vi "ciclos2.vi"() -> ()   [LabVIEW 2013]
panel:
  out "Menor":dbl
  out "Mayor":dbl
  out "Promedio":dbl
  out "Temperatura":i32(slide) scale=0.0..60.0
  # "Generar 10 temperaturas , y al final presentar la temperatura mayor , menor y la temperatura promedio"
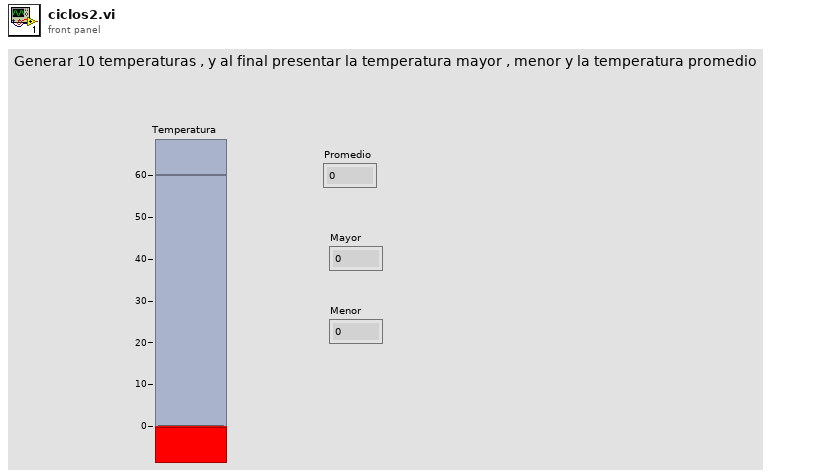
[diagram p1: front panel]
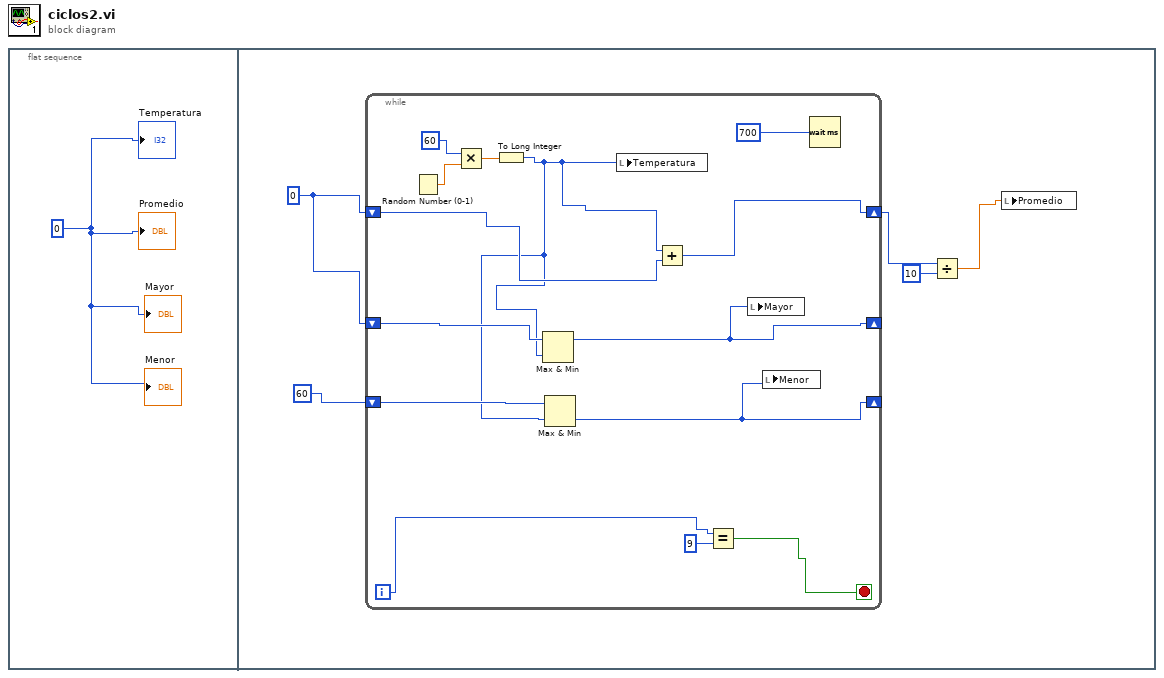
[diagram p0: block diagram]
diagram:
  n1 = flat-sequence {
    frame #0 {
      w1 = 0
      "Temperatura" <- w1
      "Promedio" <- w1
      "Mayor" <- w1
      "Menor" <- w1
    }
    frame #1 {
      w3 = 0
      n2 = while {
        shift-right: [w13] -> w6
        shift-left: w3 -> [w14]
        shift-right: [w8] -> _
        shift-left: w3 -> [w11]
        shift-right: [w7] -> _
        shift-left: 60 -> [w10]
        i -> [w20]
        stop <- w18 stop-if-true
        n3 = Random Number (0-1)() -> (number: 0 to 1=w17:dbl)
        n4 = Multiply(x=60, y=w17) -> (x*y=w15:dbl)
        n5 = To Long Integer(number=w15) -> (32bit integer=w9:i32)
        n6 = Max & Min(x=w11, y=w9) -> (max(x,y)=w8:i32)  [unwired: 1 out]
        n7 = Max & Min(x=w10, y=w9) -> (min(x,y)=w7:i32)  [unwired: 1 out]
        n8 = local write "Temperatura"(w9) -> ()
        n9 = Add(x=w9, y=w14) -> (x+y=w13:i32)
        n10 = Equal?(x=w20, y=9) -> (x = y?=w18:bool)
        n11 = local write "Mayor"(w8) -> ()
        n12 = local write "Menor"(w7) -> ()
        n13 = Wait (ms)(milliseconds to wait=700) -> ()  [unwired: 1 out]
      }
      n14 = Divide(x=w6, y=10) -> (x/y=w4:dbl)
      n15 = local write "Promedio"(w4) -> ()
    }
  }
